vi "FrecuenciasDTMF_a_CaracterTecla.vi"(1 "Min_Frecuencia":dbl, 2 "Max_Frecuencia":dbl) -> (0 "Caracter_Tecla":string)   [LabVIEW 2018]
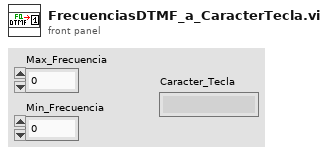
[diagram p1: front panel]
types:
  T1 = cluster{"Frecuencia_Alta":dbl, "Frecuencia_Baja":dbl, "Indicador_Tecla":dbl, "Tecla":string}[]
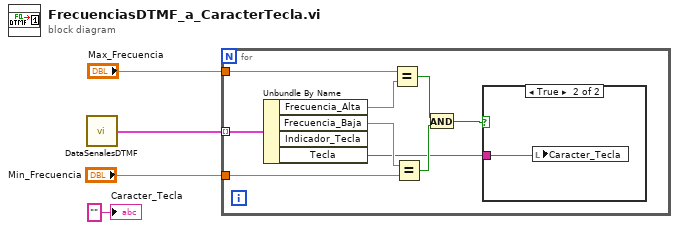
[diagram p0: block diagram]
diagram:
  n1 = call "DataSenalesDTMF.vi"() -> ("Data_Senales_DTMF"=w4:T1)  [unwired: 1 in]
  n2 = for {
    tunnel: w4 -> [w13] mode=indexing
    tunnel: "Max_Frecuencia" -> [w12]
    tunnel: "Min_Frecuencia" -> [w10]
    n3 = Unbundle By Name(w13) -> ("Frecuencia_Alta"=w11:dbl, "Frecuencia_Baja"=w9:dbl, "Tecla"=w5:string)  [unwired: 1 out]
    n4 = Equal?(x=w12, y=w11) -> (x = y?=w8:bool)
    n5 = Equal?(x=w9, y=w10) -> (x = y?=w7:bool)
    n6 = And(x=w8, y=w7) -> (x .and. y?=w6:bool)
    n7 = case shown="True" w6 {
      tunnel: w5 -> [_ w14]
      frame False {
      }
      frame True {
        n8 = local write "Caracter_Tecla"(w14) -> ()
      }
    }
  }
  "Caracter_Tecla" <- "" ("Caracter_Tecla")
